vi "Test Get Failed or Not Executed Tests Filters Passed.vi"(8 "error in (no error)":errorcluster, 11 "Result Model Result Recording Test in":refnum<class "Result Model Result Recording Test.lvclass">) -> (0 "error out":errorcluster, 3 "Result Model Result Recording Test out":refnum<class "Result Model Result Recording Test.lvclass">)   [LabVIEW 2020, in "Result Model Result Recording Test.lvclass"]
uses:
  Result Model Result Recording Test.lvclass
  source/User Interface/Result Model by Reference/Result Model by Reference.lvclass
  ae2c71b8-32bb-49d1-8500-0119bfec74ff.vi
  source/User Interface/Result Model/Tree Item Filter.ctl
  source/User Interface/Result Model/Result Model.lvclass
  source/Core/Result/Status.ctl
  source/Core/Result/Result.lvlib
  source/Core/Result/Type.ctl
  source/Core/Result/Result.ctl
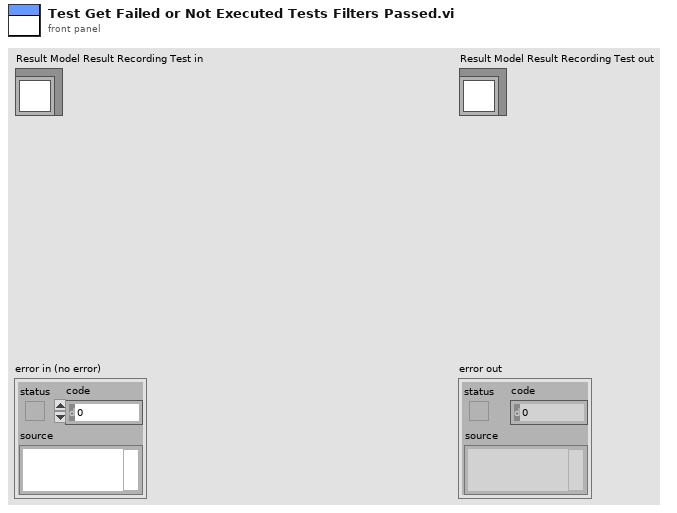
[diagram p1: front panel]
types:
  T1 = typedef "Result.lvlib/Result.ctl" = cluster{"Name":string, "Description":string, "Status":T2, "Result Type":T3, "Execution Time":dbl, "Data":cluster{"Expected":variant, "Actual":variant, "Delta":variant}}
  T2 = typedef "Result.lvlib/Status.ctl" = enum16{"", "Passed", "Failed", "Error", "Skipped", "Setup Error", "Broken", "Teardown Error"}
  T3 = typedef "Result.lvlib/Type.ctl" = enum16{"Test Case", "Test Suite", "Test Run", "Pass", "Fail", "Skip", "Pass if", "Fail if", "Pass if Error", "Fail if Error", "Pass if Equal", "Fail if Equal"}
  T4 = typedef "Result Model.lvclass/Tree Item Filter.ctl" = enum16{"All", "Only Fails", "Fails or else Not Executed"}
  T5 = cluster{"Left Cell String":string, "Child Text":string[], "Child Tag":string, "Item Indent":i32, "Child Only?":bool, "Glyph Index":i32}[]
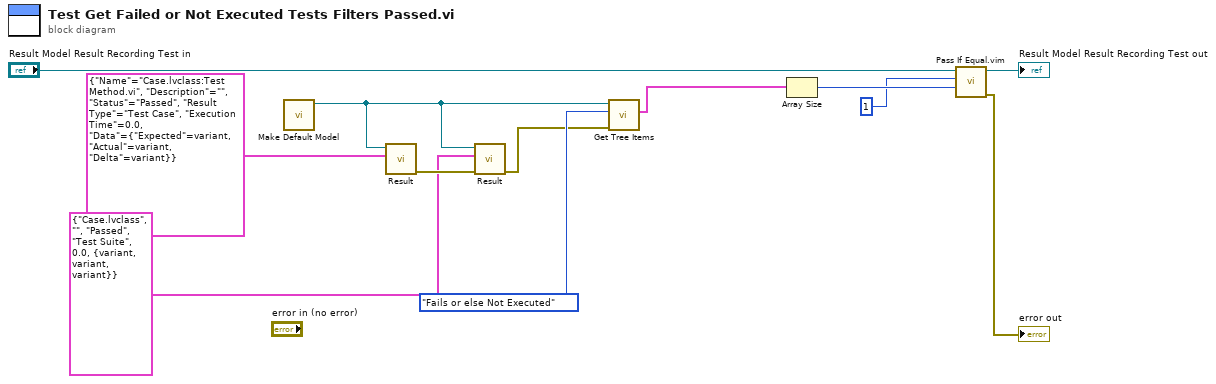
[diagram p0: block diagram]
diagram:
  n1 = call "Make Default Model.vi"() -> ("Result Model out"=w4:refnum<class "Result Model by Reference.lvclass">)  [unwired: 10 in, 1 out]
  n2 = call-dynamic "Result.vi"("Results"=T1 {"Name"="Case.lvclass:Test Method.vi", "Description"="", "Status"=enum."Passed", "Result Type"=enum."Test Case", "Execution Time"=0.0, "Data"={"Expected"=variant, "Actual"=variant, "Delta"=variant}}, "Result Model by Reference In"=w4) -> ("error out"=w3:errorcluster)  [unwired: 9 in]
  n3 = call-dynamic "Result.vi"("error in (no error)"=w3, "Results"=T1 {"Name"="Case.lvclass", "Description"="", "Status"=enum."Passed", "Result Type"=enum."Test Suite", "Execution Time"=0.0, "Data"={"Expected"=variant, "Actual"=variant, "Delta"=variant}}, "Result Model by Reference In"=w4) -> ("error out"=w2:errorcluster)  [unwired: 8 in]
  n4 = call "Get Tree Items.vi"("error in (no error)"=w2, "Filter"=Tree_Item_Filter."Fails or else Not Executed", "Result Model by Reference In"=w4) -> ("Tree Items"=w12:T5)  [unwired: 7 in, 1 out]
  n5 = Array Size(array=w12) -> (size(s)=w8:i32)
  n6 = call "Pass If Equal.vim"("Actual"=w8, "Expected"=1 ("size(s)"), "LUnit Test Case In"="Result Model Result Recording Test in") -> ("error out"=→"error out":errorcluster, "LUnit Test Case Out"=→"Result Model Result Recording Test out":refnum<class "Result Model Result Recording Test.lvclass">)  [unwired: 7 in]
